vi "Calculate Packet Timestamp Offset.vi"(0 "first packet timestamp (bytes)":u8[](array[numeric]), 5 "start trigger delay (s)":i64) -> (4 "packet timestamp offset":i64)   [LabVIEW 2023, in "GettingStarted_Gen_148X_Host.lvlib"]
uses:
  GettingStarted_Gen_148X_Host.lvlib
  <instrlib>/FlexRIO/CSI-2/v2/FPGA/Types/Raw Timestamp.ctl
  <instrlib>/FlexRIO/CSI-2/v2/Host/subVIs/Convert Raw Timestamp to LLP Packet Timestamp.vi
  <instrlib>/FlexRIO/CSI-2/v2/Host/NI CSI-2 API Host v2.lvlib
  <instrlib>/FlexRIO/CSI-2/v2/FPGA/NI CSI-2 API FPGA v2.lvlib
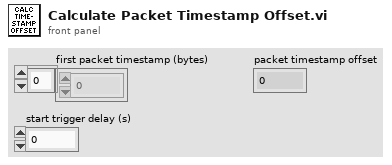
[diagram p1: front panel]
types:
  T1 = typedef "NI CSI-2 API FPGA v2.lvlib/Raw Timestamp.ctl" = cluster{"timestamp":u64, "valid":bool}
  T2 = enum16{"big-endian, network order", "native, host order", "little-endian"}
  T3 = typedef "NI CSI-2 API Host v2.lvlib/Host LLP Packet Timestamp.ctl" = cluster{"valid":bool, "count":u64, "id":T4, "metadata":u8}
  T4 = typedef "NI CSI-2 API FPGA v2.lvlib/Timestamp ID.ctl" = enum8{"SI0 LLP", "SI1 LLP", "SI2 LLP", "SI3 LLP", "SI4 LLP", "SI5 LLP", "SI6 LLP", "SI7 LLP", "SO0 LLP", "SO1 LLP", "SO2 LLP", "SO3 LLP", "SO4 LLP", "SO5 LLP", "SO6 LLP", "SO7 LLP", "Ser0 GPIO Bank", "Ser1 GPIO Bank", "Ser2 GPIO Bank", "Ser3 GPIO Bank", "Ser4 GPIO Bank", "Ser5 GPIO Bank", "Ser6 GPIO Bank", "Ser7 GPIO Bank", "Des0 GPIO Bank", "Des1 GPIO Bank", "Des2 GPIO Bank", "Des3 GPIO Bank", "Des4 GPIO Bank", "Des5 GPIO Bank", "Des6 GPIO Bank", "Des7 GPIO Bank", "User0", "User1", "User2", "User3", "User4", "User5", "User6", "User7", "User8", "User9", "User10", "User11", "User12", "User13", "User14", "User15", "User16", "User17", "User18", "User19", "User20", "User21", "User22", "User23", "User24", "User25", "User26", "User27", "User28", "User29", "User30", "User31"}
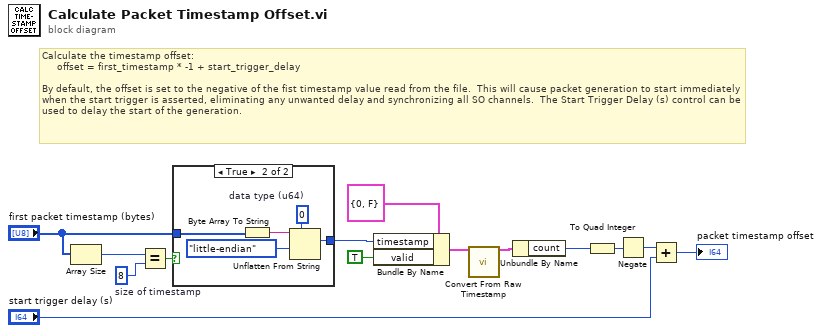
[diagram p0: block diagram]
diagram:
  w1 = 8  # size of timestamp
  # "Calculate the timestamp offset:\n     offset = first_timestamp * -1 + start_trigger_delay\n\nBy default, the offset is set to the negative of the fist timestamp value read from the file.  This will cause packet generation to start immediately when the start trigger is asserted, eliminating any unwanted delay and synchronizing all SO channels.  The Start Trigger Delay (s) control can be used to delay the start of the generation."
  n1 = Array Size(array="first packet timestamp (bytes)") -> (size(s)=w3:i32)
  n2 = Equal?(x=w3, y=w1) -> (x = y?=w4:bool)
  n3 = case shown="True" w4 {
    tunnel: [_ w16] -> w13
    tunnel: "first packet timestamp (bytes)" -> [_ w15]
    frame False {
    }
    frame True {
      w17 = u64 0  # data type (u64)
      n4 = Byte Array To String(unsigned byte array=w15) -> (string=w19:string)
      n5 = Unflatten From String(type=w17, binary string=w19, byte order (0:big-endian, network order)=T2."little-endian") -> (value=w16:u64)  [unwired: 2 in, 2 out]
    }
  }
  n6 = Bundle By Name(cluster=T1 {"timestamp"=0, "valid"=FALSE} ("raw timestamp"), "timestamp"=w13, "valid"=TRUE) -> (w11:T1)
  n7 = call-poly <instrlib>:"Convert From Raw Timestamp.vi"("raw timestamp"=w11) -> ("llp packet timestamp"=w10:T3)  [unwired: 14 in]
  n8 = Unbundle By Name(w10) -> ("count"=w7:u64)
  n9 = To Quad Integer(1:w7) -> (0:w9:i64)
  n10 = Negate(x=w9) -> (-x=w8:i64)
  n11 = Add(x=w8, y="start trigger delay (s)") -> (x+y=→"packet timestamp offset":i64)
